vi "Reposition Front Panel.vi"(11 "reference":refnum<vi>) -> (0 "error out":errorcluster)   [LabVIEW 2017]
uses:
  <vilib>/Utility/miscctls.llb/LVRectTypeDef.ctl
  <vilib>/Utility/miscctls.llb/LVPointTypeDef.ctl
panel:
  out "Display:Primary Workspace":T1
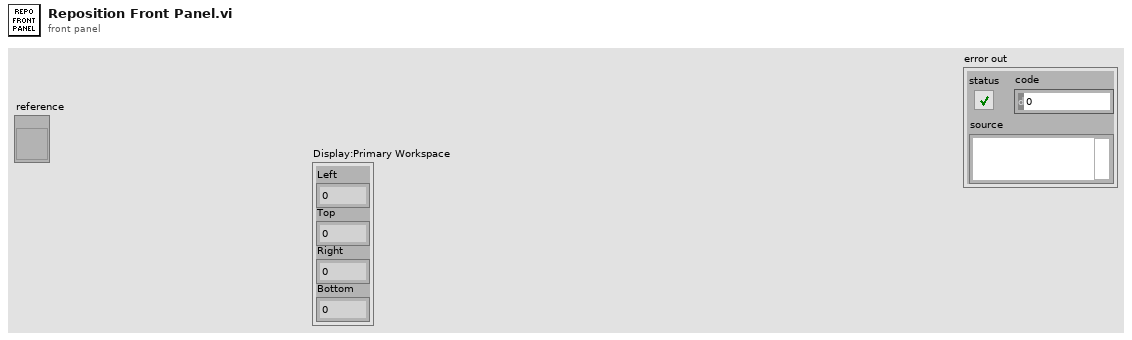
[diagram p1: front panel]
types:
  T1 = typedef "LVRectTypeDef.ctl" = cluster{"Left":i16, "Top":i16, "Right":i16, "Bottom":i16}
  T2 = typedef "LVPointTypeDef.ctl" = cluster{"Horizontal":i16, "Vertical":i16}
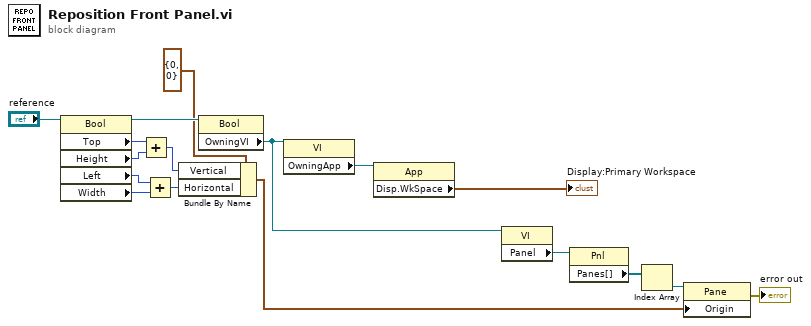
[diagram p0: block diagram]
diagram:
  n1 = property class="Bool"(reference="reference") -> (reference out=w13:refnum<vi>, "Top"=w17:i32, "Height"=w16:u32, "Left"=w15:i32, "Width"=w14:u32)  [unwired: 1 in, 1 out]
  n2 = Add(x=w17, y=w16) -> (x+y=w12:u32)
  n3 = Add(x=w15, y=w14) -> (x+y=w11:u32)
  n4 = Bundle By Name(cluster=T2 {"Horizontal"=0, "Vertical"=0} ("Origin"), "Vertical"=w12, "Horizontal"=w11) -> (w3:T2)
  n5 = property on="Property Node" class="Bool"(reference=w13) -> ("OwningVI"=w9:refnum<vi>)  [unwired: 1 in, 2 out]
  n6 = property on="Property Node" class="VI"(reference=w9) -> ("OwningApp"=w10:refnum<vi>)  [unwired: 1 in, 2 out]
  n7 = property on="Property Node" class="App"(reference=w10) -> ("Disp.WkSpace"=→"Display:Primary Workspace":T1)  [unwired: 1 in, 2 out]
  n8 = property on="Property Node" class="VI"(reference=w9) -> ("Panel"=w7:refnum<vi>)  [unwired: 1 in, 2 out]
  n9 = property on="Property Node" class="Pnl"(reference=w7) -> ("Panes[]"=w6:refnum<vi>[])  [unwired: 1 in, 2 out]
  n10 = Index Array(array=w6) -> (element=w5:refnum<vi>)  [unwired: 1 in]
  n11 = property on="Property Node" class="Pane"(reference=w5, "Origin"=w3) -> (error out=→"error out":errorcluster)  [unwired: 1 in, 1 out]
